vi "stop.vi"(0 "VISA resource name":refnum<visa-resource-name>, 3 "error in (no error)":errorcluster) -> (6 "VISA resource name out":refnum<visa-resource-name>, 9 "Error out":errorcluster)   [LabVIEW 2017]
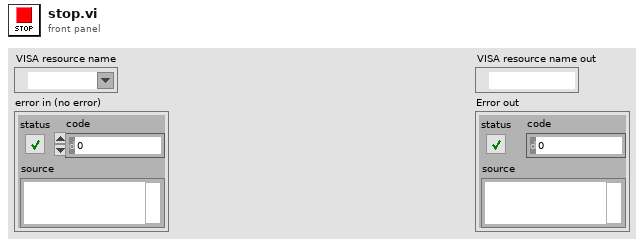
[diagram p1: front panel]
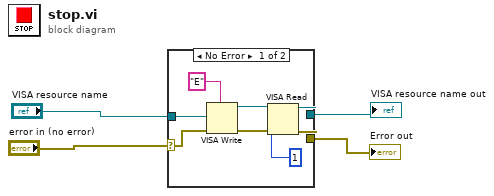
[diagram p0: block diagram]
diagram:
  n1 = case shown="No Error" "error in (no error)" {
    selector: "error in (no error)" -> [w10 w13]
    tunnel: "VISA resource name" -> [w11 w14]
    tunnel: [w6 w14] -> w2
    tunnel: [w5 w13] -> w1
    frame No Error {
      n2 = VISA Write(VISA resource name=w11, write buffer="E", error in (no error)=w10) -> (VISA resource name out=w7:refnum<visa-resource-name>, error out=w9:errorcluster)  [unwired: 1 out]
      n3 = VISA Read(VISA resource name=w7, byte count=u32 1, error in (no error)=w9) -> (VISA resource name out=w6:refnum<visa-resource-name>, error out=w5:errorcluster)  [unwired: 2 out]
    }
    frame Error {
    }
  }
  "VISA resource name out" <- w2
  "Error out" <- w1
